vi "作业3跑马灯条件结构.vi"() -> ()   [LabVIEW 2022 SP3]
panel:
  in  "停止":bool
  in  "滑动杆":dbl(slide) scale=0.0..10.0
  out "布尔 5":bool
  out "布尔 4":bool
  out "布尔 3":bool
  out "布尔 2":bool
  out "布尔":bool
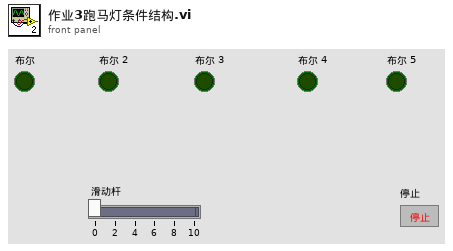
[diagram p1: front panel]
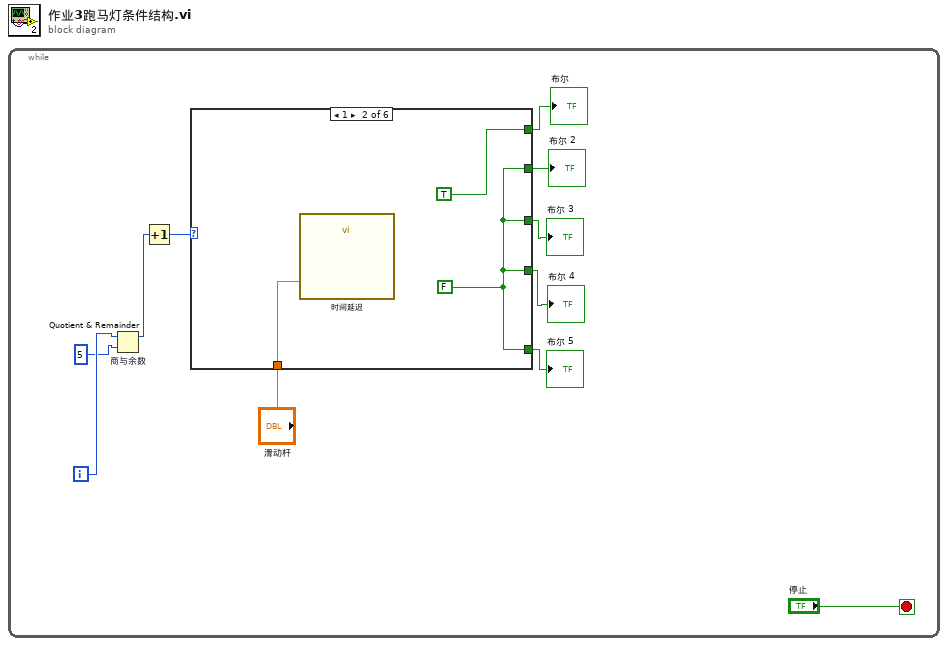
[diagram p0: block diagram]
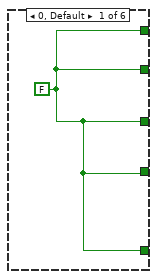
[diagram p2: hidden frame]
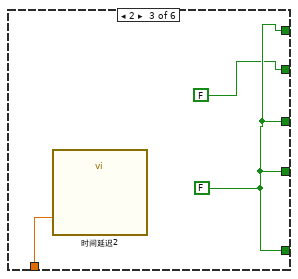
[diagram p3: hidden frame]
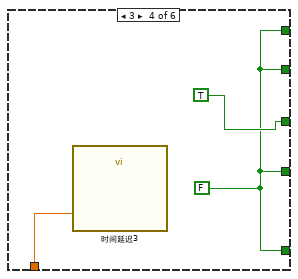
[diagram p4: hidden frame]
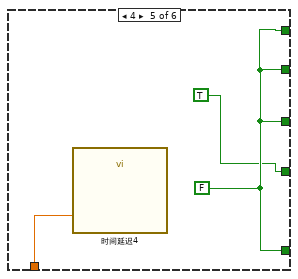
[diagram p5: hidden frame]
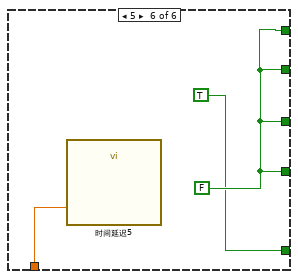
[diagram p6: hidden frame]
diagram:
  n1 = while {
    i -> [w11]
    stop <- "停止" stop-if-true
    n2 = Quotient & Remainder "商与余数"(x=w11, y=5) -> (x-y*floor(x/y)=w3:i32)  [unwired: 1 out]
    n3 = Increment(x=w3) -> (x+1=w4:i32)
    n4 = case shown="1" w4 {
      tunnel: [w12 TRUE w18 w20 w24 w27] -> w9
      tunnel: [w12 w14 FALSE w20 w24 w27] -> w8
      tunnel: [w12 w14 w18 TRUE w24 w27] -> w7
      tunnel: [w12 w14 w18 w20 TRUE w27] -> w6
      tunnel: [w12 w14 w18 w20 w24 TRUE] -> w5
      tunnel: "滑动杆" -> [_ w13 w16 w19 w22 w25]
      frame 0, Default {
        w12 = FALSE
      }
      frame 1 {
        w14 = FALSE
        n5 = call "时间延迟"("Delay Time (s)"=w13) -> ()  [unwired: 10 in, 1 out]
      }
      frame 2 {
        w18 = FALSE
        n6 = call "时间延迟2"("Delay Time (s)"=w16) -> ()  [unwired: 10 in, 1 out]
      }
      frame 3 {
        w20 = FALSE
        n7 = call "时间延迟3"("Delay Time (s)"=w19) -> ()  [unwired: 10 in, 1 out]
      }
      frame 4 {
        w24 = FALSE
        n8 = call "时间延迟4"("Delay Time (s)"=w22) -> ()  [unwired: 10 in, 1 out]
      }
      frame 5 {
        w27 = FALSE
        n9 = call "时间延迟5"("Delay Time (s)"=w25) -> ()  [unwired: 10 in, 1 out]
      }
    }
    "布尔 5" <- w5
    "布尔" <- w9
    "布尔 2" <- w8
    "布尔 3" <- w7
    "布尔 4" <- w6
  }
